vi "SequenceSaver.vi"(11 "Sequence Storer":T1[][](array[typedef])=[[{"Position"={"x"=0.000648543, "y"=-0.00013342599999999986, "z"=0.0}, "Intensity"=1.0, "Vortex Charge"=0, "Phase"=0.0, "NA Position"={"x"=0.0, "y"=0.0, "r"=1.0}, "Line Trapping"={"Vector"={"x"=0.0, "y"=0.0, "z"=0.0}, "Phase Gradient"=0.0}, "Amplitude Correction"=0.0}, {"Position"={"x"=0.0001674748340595137, "y"=-0.0001324825534959771, "z"=0.0}, "Intensity"=1.0, "Vortex Charge"=0, "Phase"=0.0, "NA Position"={"x"=0.0, "y"=0.0, "r"=1.0}, "Line Trapping"={"Vector"={"x"=0.0, "y"=0.0, "z"=0.0}, "Phase Gradient"=0.0}, "Amplitude Correction"=0.0}], [{"Position"={"x"=0.000648543, "y"=-6.309774702800111e-05, "z"=0.0}, "Intensity"=1.0, "Vortex Charge"=0, "Phase"=0.0, "NA Position"={"x"=0.0, "y"=0.0, "r"=1.0}, "Line Trapping"={"Vector"={"x"=0.0, "y"=0.0, "z"=0.0}, "Phase Gradient"=0.0}, "Amplitude Correction"=0.0}, {"Position"={"x"=0.0001674748340595137, "y"=-6.215430052397834e-05, "z"=0.0}, "Intensity"=1.0, "Vortex Charge"=0, "Phase"=0.0, "NA Position"={"x"=0.0, "y"=0.0, "r"=1.0}, "Line Trapping"={"Vector"={"x"=0.0, "y"=0.0, "z"=0.0}, "Phase Gradient"=0.0}, "Amplitude Correction"=0.0}], [{"Position"={"x"=0.000648543, "y"=7.230505943997632e-06, "z"=0.0}, "Intensity"=1.0, "Vortex Charge"=0, "Phase"=0.0, "NA Position"={"x"=0.0, "y"=0.0, "r"=1.0}, "Line Trapping"={"Vector"={"x"=0.0, "y"=0.0, "z"=0.0}, "Phase Gradient"=0.0}, "Amplitude Correction"=0.0}, {"Position"={"x"=0.0001674748340595137, "y"=8.1739524480204e-06, "z"=0.0}, "Intensity"=1.0, "Vortex Charge"=0, "Phase"=0.0, "NA Position"={"x"=0.0, "y"=0.0, "r"=1.0}, "Line Trapping"={"Vector"={"x"=0.0, "y"=0.0, "z"=0.0}, "Phase Gradient"=0.0}, "Amplitude Correction"=0.0}], [{"Position"={"x"=0.000648543, "y"=7.755875891599632e-05, "z"=0.0}, "Intensity"=1.0, "Vortex Charge"=0, "Phase"=0.0, "NA Position"={"x"=0.0, "y"=0.0, "r"=1.0}, "Line Trapping"={"Vector"={"x"=0.0, "y"=0.0, "z"=0.0}, "Phase Gradient"=0.0}, "Amplitude Correction"=0.0}, {"Position"={"x"=0.0001674748340595137, "y"=7.850220542001909e-05, "z"=0.0}, "Intensity"=1.0, "Vortex Charge"=0, "Phase"=0.0, "NA Position"={"x"=0.0, "y"=0.0, "r"=1.0}, "Line Trapping"={"Vector"={"x"=0.0, "y"=0.0, "z"=0.0}, "Phase Gradient"=0.0}, "Amplitude Correction"=0.0}], [{"Position"={"x"=0.000648543, "y"=0.000147887011887995, "z"=0.0}, "Intensity"=1.0, "Vortex Charge"=0, "Phase"=0.0, "NA Position"={"x"=0.0, "y"=0.0, "r"=1.0}, "Line Trapping"={"Vector"={"x"=0.0, "y"=0.0, "z"=0.0}, "Phase Gradient"=0.0}, "Amplitude Correction"=0.0}, {"Position"={"x"=0.0001674748340595137, "y"=0.00014883045839201778, "z"=0.0}, "Intensity"=1.0, "Vortex Charge"=0, "Phase"=0.0, "NA Position"={"x"=0.0, "y"=0.0, "r"=1.0}, "Line Trapping"={"Vector"={"x"=0.0, "y"=0.0, "z"=0.0}, "Phase Gradient"=0.0}, "Amplitude Correction"=0.0}], [{"Position"={"x"=0.000648543, "y"=0.00021821526485999376, "z"=0.0}, "Intensity"=1.0, "Vortex Charge"=0, "Phase"=0.0, "NA Position"={"x"=0.0, "y"=0.0, "r"=1.0}, "Line Trapping"={"Vector"={"x"=0.0, "y"=0.0, "z"=0.0}, "Phase Gradient"=0.0}, "Amplitude Correction"=0.0}, {"Position"={"x"=0.0001674748340595137, "y"=0.00021915871136401653, "z"=0.0}, "Intensity"=1.0, "Vortex Charge"=0, "Phase"=0.0, "NA Position"={"x"=0.0, "y"=0.0, "r"=1.0}, "Line Trapping"={"Vector"={"x"=0.0, "y"=0.0, "z"=0.0}, "Phase Gradient"=0.0}, "Amplitude Correction"=0.0}], [{"Position"={"x"=0.000648543, "y"=0.0002885435178319925, "z"=0.0}, "Intensity"=1.0, "Vortex Charge"=0, "Phase"=0.0, "NA Position"={"x"=0.0, "y"=0.0, "r"=1.0}, "Line Trapping"={"Vector"={"x"=0.0, "y"=0.0, "z"=0.0}, "Phase Gradient"=0.0}, "Amplitude Correction"=0.0}, {"Position"={"x"=0.0001674748340595137, "y"=0.00028948696433601527, "z"=0.0}, "Intensity"=1.0, "Vortex Charge"=0, "Phase"=0.0, "NA Position"={"x"=0.0, "y"=0.0, "r"=1.0}, "Line Trapping"={"Vector"={"x"=0.0, "y"=0.0, "z"=0.0}, "Phase Gradient"=0.0}, "Amplitude Correction"=0.0}], [{"Position"={"x"=0.000648543, "y"=0.0003588717708039912, "z"=0.0}, "Intensity"=1.0, "Vortex Charge"=0, "Phase"=0.0, "NA Position"={"x"=0.0, "y"=0.0, "r"=1.0}, "Line Trapping"={"Vector"={"x"=0.0, "y"=0.0, "z"=0.0}, "Phase Gradient"=0.0}, "Amplitude Correction"=0.0}, {"Position"={"x"=0.0001674748340595137, "y"=0.00035981521730801396, "z"=0.0}, "Intensity"=1.0, "Vortex Charge"=0, "Phase"=0.0, "NA Position"={"x"=0.0, "y"=0.0, "r"=1.0}, "Line Trapping"={"Vector"={"x"=0.0, "y"=0.0, "z"=0.0}, "Phase Gradient"=0.0}, "Amplitude Correction"=0.0}], [{"Position"={"x"=0.000648543, "y"=0.0004292000237759899, "z"=0.0}, "Intensity"=1.0, "Vortex Charge"=0, "Phase"=0.0, "NA Position"={"x"=0.0, "y"=0.0, "r"=1.0}, "Line Trapping"={"Vector"={"x"=0.0, "y"=0.0, "z"=0.0}, "Phase Gradient"=0.0}, "Amplitude Correction"=0.0}, {"Position"={"x"=0.0001674748340595137, "y"=0.00043014347028001265, "z"=0.0}, "Intensity"=1.0, "Vortex Charge"=0, "Phase"=0.0, "NA Position"={"x"=0.0, "y"=0.0, "r"=1.0}, "Line Trapping"={"Vector"={"x"=0.0, "y"=0.0, "z"=0.0}, "Phase Gradient"=0.0}, "Amplitude Correction"=0.0}], [{"Position"={"x"=0.000648543, "y"=0.0004995282767479886, "z"=0.0}, "Intensity"=1.0, "Vortex Charge"=0, "Phase"=0.0, "NA Position"={"x"=0.0, "y"=0.0, "r"=1.0}, "Line Trapping"={"Vector"={"x"=0.0, "y"=0.0, "z"=0.0}, "Phase Gradient"=0.0}, "Amplitude Correction"=0.0}, {"Position"={"x"=0.0001674748340595137, "y"=0.0005004717232520114, "z"=0.0}, "Intensity"=1.0, "Vortex Charge"=0, "Phase"=0.0, "NA Position"={"x"=0.0, "y"=0.0, "r"=1.0}, "Line Trapping"={"Vector"={"x"=0.0, "y"=0.0, "z"=0.0}, "Phase Gradient"=0.0}, "Amplitude Correction"=0.0}]] {"Amplitude Correction" step=0.1; "Line Trapping"."Phase Gradient" step=0.05; "Line Trapping"."Vector"."x" step=1e-06 format="%#_6p"; "Line Trapping"."Vector"."y" step=1e-06 format="%#_6p"; "Line Trapping"."Vector"."z" step=1e-06 format="%#_6p"; "NA Position"."r" step=1e-06; "NA Position"."y" step=1e-06; "NA Position"."x" step=1e-06; "Position"."z" step=1e-06; "Position"."y" step=1e-06; "Position"."x" step=1e-06; "Phase" step=0.7753; "Intensity" step=0.1}) -> (3 "Sequence Storer 2":T1[][](array[typedef]) {"Amplitude Correction" step=0.1; "Line Trapping"."Phase Gradient" step=0.05; "Line Trapping"."Vector"."x" step=1e-06 format="%#_6p"; "Line Trapping"."Vector"."y" step=1e-06 format="%#_6p"; "Line Trapping"."Vector"."z" step=1e-06 format="%#_6p"; "NA Position"."r" step=1e-06; "NA Position"."y" step=1e-06; "NA Position"."x" step=1e-06; "Position"."z" step=1e-06; "Position"."y" step=1e-06; "Position"."x" step=1e-06; "Phase" step=0.7753; "Intensity" step=0.1})   [LabVIEW 2015]
uses:
  spot.ctl
  line_trapping.ctl
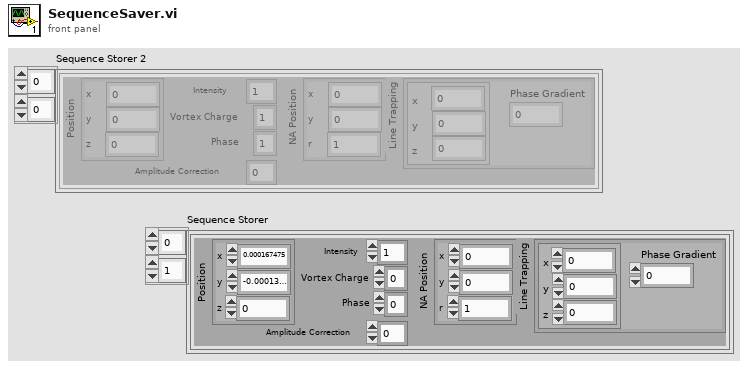
[diagram p1: front panel]
types:
  T1 = typedef "spot.ctl" = cluster{"Position":cluster{"x":dbl, "y":dbl, "z":dbl}, "Intensity":dbl, "Vortex Charge":i8, "Phase":dbl, "NA Position":cluster{"x":dbl, "y":dbl, "r":dbl}, "Line Trapping":T2, "Amplitude Correction":dbl}
  T2 = typedef "line_trapping.ctl" = cluster{"Vector":cluster{"x":dbl, "y":dbl, "z":dbl}, "Phase Gradient":dbl}
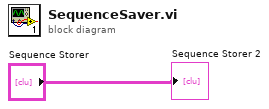
[diagram p0: block diagram]
diagram:
  "Sequence Storer 2" <- "Sequence Storer"
